vi "AMZ_S3_APIHLP_Get XML Tags value.vi"(7 "Tag name":string, 8 "error in (no error)":errorcluster, 11 "XML String in":string) -> (0 "error out":errorcluster, 2 "Remaining string":string, 3 "Value":string)   [LabVIEW 2015, in "LV Interface for Amazon S3.lvlib"]
doc: "Returns everything in between the first occurence of the specified tag's opening and closing brackets.\nNote! This VI will return nested elements as well!\nIt also returns remaining string, so you can use it in a loop with a shift register passing back the remaining string."
uses:
  LV Interface for Amazon S3.lvlib
  <vilib>/regexp/Match Regular Expression.xnode
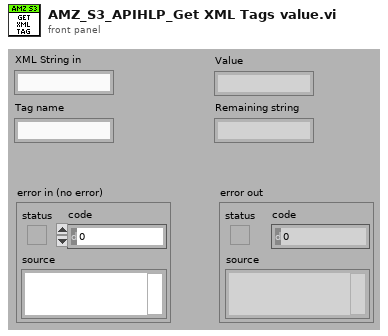
[diagram p1: front panel]
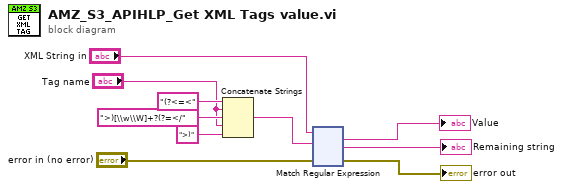
[diagram p0: block diagram]
diagram:
  n1 = Concatenate Strings("(?<=<", "Tag name", ">)[\\w\\W]+?(?=</", "Tag name", ">)") -> (w4:string)
  n2 = xnode "Match Regular Expression"("input string"="XML String in", "regular expression"=w4, "error in"="error in (no error)") -> ("whole match"=→"Value":string, "after match"=→"Remaining string":string, "error out"=→"error out":errorcluster)  [unwired: 3 in, 2 out]
